vi "VIP_Pre-Uninstall Custom Action.vi"(10 "Variant":variant) -> (0 "error out":errorcluster)   [LabVIEW 2021]
uses:
  <resource>/dialog/lvconfig.llb/LV Config Read String.vi
  <userlib>/_OpenG.lib/file/file.llb/Convert File Extension (Path)__ogtk.vi
  <userlib>/_OpenG.lib/lvzip/lvzip.llb/subVI/ZLIB Extract All Files To Dir (Path)__ogtk.vi
  <vilib>/regexp/Match Regular Expression.xnode
  <userlib>/_OpenG.lib/file/file.llb/openg_file.lvlib
panel:
  # "pre uninstall"
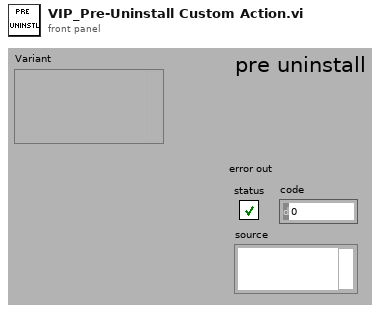
[diagram p1: front panel]
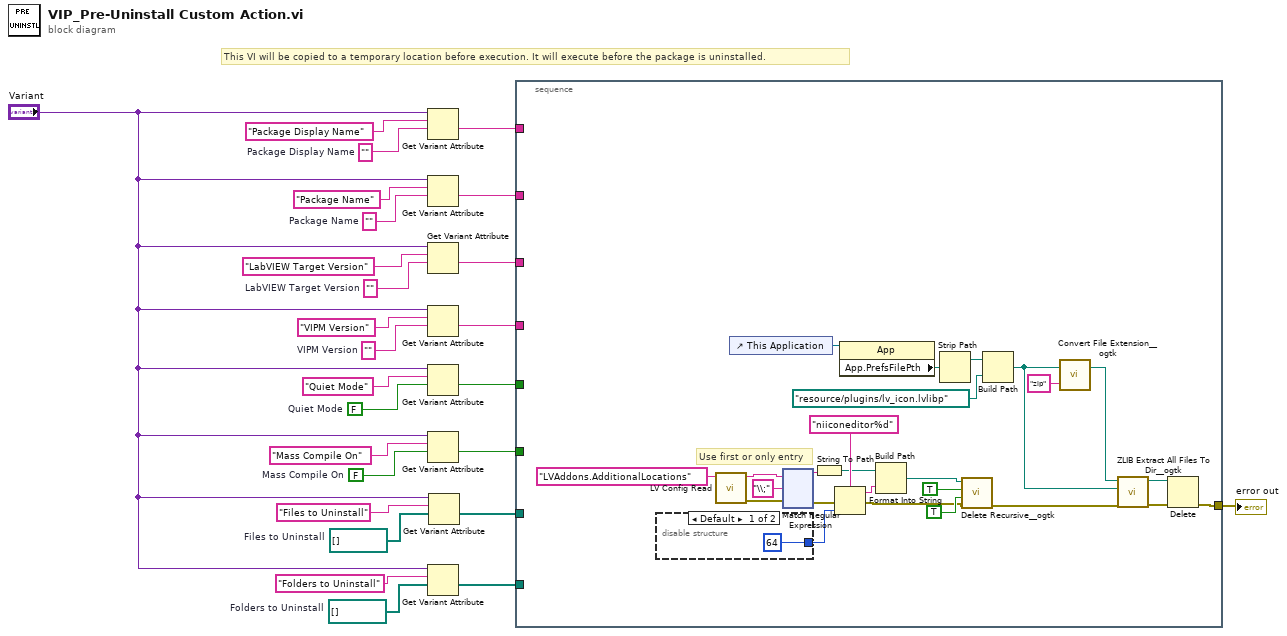
[diagram p0: block diagram]
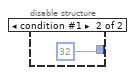
[diagram p2: hidden frame]
diagram:
  w11 = path[] []  # Folders to Uninstall
  w14 = path[] []  # Files to Uninstall
  w15 = FALSE  # Mass Compile On
  w16 = ""  # Package Display Name
  w17 = FALSE  # Quiet Mode
  w20 = ""  # VIPM Version
  w22 = ""  # LabVIEW Target Version
  w24 = ""  # Package Name
  # "This VI will be copied to a temporary location before execution. It will execute before the package is uninstalled."
  n1 = Get Variant Attribute(Variant="Variant", name="Package Display Name", default value (empty Variant)=w16) -> (value=w9:string)  [unwired: 1 in, 3 out]
  n2 = Get Variant Attribute(Variant="Variant", name="Package Name", default value (empty Variant)=w24) -> (value=w8:string)  [unwired: 1 in, 3 out]
  n3 = Get Variant Attribute(Variant="Variant", name="LabVIEW Target Version", default value (empty Variant)=w22) -> (value=w7:string)  [unwired: 1 in, 3 out]
  n4 = Get Variant Attribute(Variant="Variant", name="VIPM Version", default value (empty Variant)=w20) -> (value=w6:string)  [unwired: 1 in, 3 out]
  n5 = Get Variant Attribute(Variant="Variant", name="Quiet Mode", default value (empty Variant)=w17) -> (value=w5:bool)  [unwired: 1 in, 3 out]
  n6 = Get Variant Attribute(Variant="Variant", name="Mass Compile On", default value (empty Variant)=w15) -> (value=w4:bool)  [unwired: 1 in, 3 out]
  n7 = Get Variant Attribute(Variant="Variant", name="Folders to Uninstall", default value (empty Variant)=w11) -> (value=w2:path[])  [unwired: 1 in, 3 out]
  n8 = Get Variant Attribute(Variant="Variant", name="Files to Uninstall", default value (empty Variant)=w14) -> (value=w3:path[])  [unwired: 1 in, 3 out]
  n9 = stacked-sequence {
    tunnel: w9 -> [_]
    tunnel: w8 -> [_]
    tunnel: w7 -> [_]
    tunnel: w6 -> [_]
    tunnel: w5 -> [_]
    tunnel: w4 -> [_]
    tunnel: w3 -> [_]
    tunnel: w2 -> [_]
    tunnel: [w27] -> w1
    frame #0 {
      # "Use first or only entry"
      n10 = disable-structure shown="Default" {
        disable-tunnel: [64 ("code") 32 ("code")] -> w47
        frame condition #0 (active) {
        }
        frame condition #1 {
        }
      }
      n11 = call-poly <resource>:"LV Config Read.vi"("key"="LVAddons.AdditionalLocations") -> ("error out"=w48:errorcluster, "value"=w46:string)  [unwired: 4 in, 1 out]
      n12 = control-ref of="This Application"() -> (w37:refnum<vi>)
      n13 = xnode "Match Regular Expression"("input string"=w46, "regular expression"="\\;", "error in"=w48) -> ("before match"=w41:string, "error out"=w49:errorcluster)  [unwired: 3 in, 3 out]
      n14 = String To Path(string=w41) -> (path=w40:path)
      n15 = Format Into String(format string="niiconeditor%d", error in=w49, w47) -> (resulting string=w39:string, error out=w42:errorcluster)  [unwired: 1 in]
      n16 = property class="App"(reference=w37) -> ("App.PrefsFilePth"=w34:path)  [unwired: 1 in, 2 out]
      n17 = Build Path(base path=w40, name or relative path=w39) -> (appended path=w38:path)
      n18 = Strip Path(path=w34) -> (stripped path=w36:path)  [unwired: 1 out]
      n19 = call <userlib>:"Delete Recursive__ogtk.vi"("error in (no error)"=w42, "Ignore Read-Only? (FALSE)"=TRUE, "Recursive? (FALSE)"=TRUE, "Path"=w38) -> ("error out"=w29:errorcluster)  [unwired: 6 in, 1 out]
      n20 = Build Path(base path=w36, name or relative path=path "resource/plugins/lv_icon.lvlibp") -> (appended path=w28:path)
      n21 = call-poly <userlib>:"Convert File Extension__ogtk.vi"("new ending (none)"="zip", "file name"=w28) -> ("new filename"=w32:path)  [unwired: 1 out]
      n22 = call-poly <userlib>:"ZLIB Extract All Files To Dir__ogtk.vi"("error in (no error)"=w29, "destination directory (archive name without ending)"=w28, "archive name (file dialog)"=w32) -> ("error out"=w31:errorcluster, "archive name out"=w30:path)  [unwired: 6 in, 1 out]
      n23 = Delete(path (use dialog)=w30, error in=w31) -> (error out=w27:errorcluster)  [unwired: 3 in, 2 out]
    }
  }
  "error out" <- w1
